vi "Coord Straight Line Move.vi"() -> ()   [LabVIEW 2014]
uses:
  <vilib>/Motion/plugins/PluginFramework/nismSDIFramework.SetFrameworkMode.single.vi
  <vilib>/Motion/PropertyNodes/nimc.createStraightLineMoveInstance.coordinate.vi
  <vilib>/Motion/PropertyNodes/nimc.destroyInterfaceInstance.vi
  <resource>/objmgr/nimotion.rc
  SDI Plug-in - Delta ASDA.lvclass
panel:
  in  "Axis 2":refnum<k21>="Axis 2"
  in  "Axis":refnum<k21>="Axis 1"
  in  "Coordinate Space":refnum<k21>="Coordinate Space 1"
  in  "Position":dbl[](array[numeric])=[1000.0, 2000.0]
  in  "Move Mode":i32(ring)=10551344 items=["Absolute"=10551337, "Relative"=10551344, "Relative To Capture"=10551345, "Velocity"=10551346]
  in  "Acceleration":dbl=10000.0
  in  "Velocity":dbl=1000.0
  out "error out":errorcluster
  out "?":T1(graph)
  in  "Stop Move":bool
  in  "Start Move":bool
  in  "stop":bool
  # "Notes: \n1. This example uses preconfigured settings that may not be appropriate for your motion system. Review and update the axis settings using the Axis Configuration dialog box. Right-click each axis and select Properties to open the Axis Configuration dialog box. \n2. Running this example automatically activates all axes. Disable the \"Enable Drive on Transition to Active Mode\" option on the General Settings page of the Axis Configuration dialog box to prevent axes from activating when the VI runs.\n3. This example uses the default smoothing value to automatically calculate deceleration and jerk values. To specify these move constraints, add them to the move property node.\n\nFor information about using this example in an actual motion system, refer to ni.com/info and enter Info Code nismex."
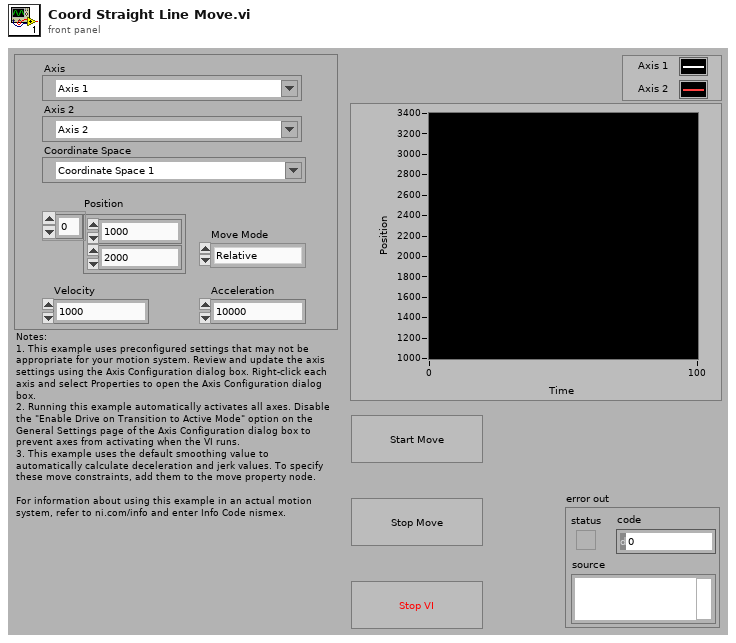
[diagram p1: front panel]
types:
  T1 = cluster{"Commanded Pos.[][0]":dbl, "Commanded Pos.[][1]":dbl}
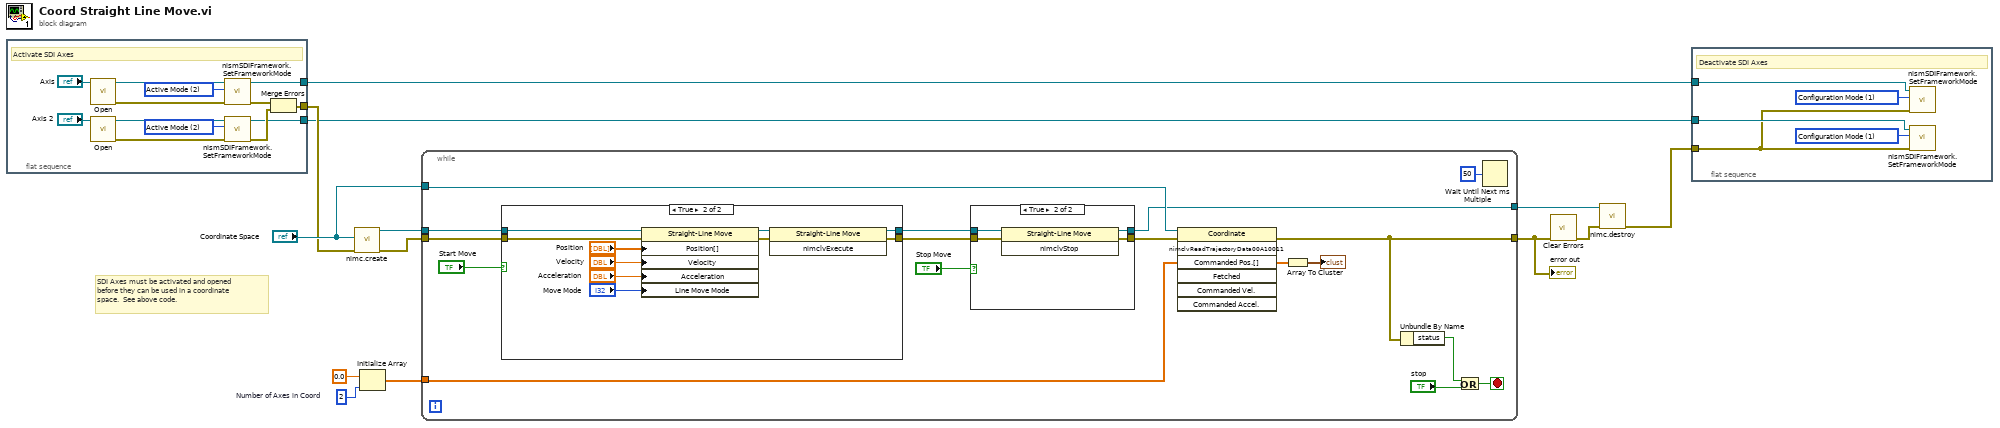
[diagram p0: block diagram]
diagram:
  w6 = 2  # Number of Axes in Coord
  # "SDI Axes must be activated and opened\nbefore they can be used in a coordinate\nspace.  See above code."
  n1 = flat-sequence {
    tunnel: [w16] -> w4
    tunnel: [w15] -> w3
    tunnel: [w14] -> w2
    frame #0 {
      w19 = 2 items=["Configuration Mode"=1, "Active Mode"=2] ("mode (Active Mode)")
      w26 = 2 items=["Configuration Mode"=1, "Active Mode"=2] ("mode (Active Mode)")
      # "Activate SDI Axes"
      n2 = call "Open.vi"("Axis"="Axis") -> ("error out"=w24:errorcluster, "Base Axis Out"=w25:refnum<class "nismPluginAxisBaseClass.lvclass">)  [unwired: 9 in]
      n3 = call "Open.vi"("Axis"="Axis 2") -> ("error out"=w21:errorcluster, "Base Axis Out"=w20:refnum<class "nismPluginAxisBaseClass.lvclass">)  [unwired: 9 in]
      n4 = call-poly <vilib>:"nismSDIFramework.SetFrameworkMode.vi"("error in (no error)"=w24, "mode (Active Mode)"=w26, "Base Axis In"=w25) -> ("error out"=w18:errorcluster, "Base Axis Out"=w15:refnum<class "nismPluginAxisBaseClass.lvclass">)  [unwired: 7 in]
      n5 = call-poly <vilib>:"nismSDIFramework.SetFrameworkMode.vi"("error in (no error)"=w21, "mode (Active Mode)"=w19, "Base Axis In"=w20) -> ("error out"=w17:errorcluster, "Base Axis Out"=w14:refnum<class "nismPluginAxisBaseClass.lvclass">)  [unwired: 7 in]
      n6 = Merge Errors(w18, w17) -> (w16:errorcluster)
    }
  }
  n7 = call-poly <vilib>:"nimc.create.vi"("error in"=w4, "coordinate"="Coordinate Space") -> ("error out"=w12:errorcluster, "line"=w13:refnum<k20>)  [unwired: 7 in, 1 out]
  n8 = Initialize Array(0.0 ("element"), w6) -> (w5:dbl[])
  n9 = while {
    tunnel: w13 -> [w43]
    tunnel: w12 -> [w42]
    tunnel: "Coordinate Space" -> [w34]
    tunnel: [w31] -> w9
    tunnel: [w30] -> w11
    tunnel: w5 -> [w29]
    stop <- w33 stop-if-true
    n10 = case shown="True" "Start Move" {
      tunnel: w43 -> [w51 w61]
      tunnel: w42 -> [w50 w58]
      tunnel: [w50 w57] -> w37
      tunnel: [w51 w56] -> w36
      frame False {
      }
      frame True {
        n11 = property class="Straight-Line Move"(reference=w61, error in=w58, "Position[]"="Position", "Velocity"="Velocity", "Acceleration"="Acceleration", "Line Move Mode"="Move Mode") -> (reference out=w60:refnum<k20>, error out=w59:errorcluster)
        n12 = invoke class="Straight-Line Move" method="nimclvExecute"(reference=w60, error in=w59) -> (reference out=w56:refnum<k20>, error out=w57:errorcluster)  [unwired: 1 in, 1 out]
      }
    }
    n13 = case shown="True" "Stop Move" {
      tunnel: w37 -> [w45 w48]
      tunnel: w36 -> [w44 w49]
      tunnel: [w45 w47] -> w35
      tunnel: [w44 w46] -> w30
      frame False {
      }
      frame True {
        n14 = invoke class="Straight-Line Move" method="nimclvStop"(reference=w49, error in=w48) -> (reference out=w46:refnum<k20>, error out=w47:errorcluster)  [unwired: 1 in, 1 out]
      }
    }
    n15 = invoke class="Coordinate" method="nimclvReadTrajectoryData00A10011"(reference=w34, error in=w35, "Commanded Pos.[]"=w29) -> (error out=w31:errorcluster, "Commanded Pos.[]"=w28:dbl[])  [unwired: 4 in, 5 out]
    n16 = Array To Cluster(array=w28) -> (cluster=→"?":T1)
    n17 = Unbundle By Name(w31) -> ("status"=w32:bool)
    n18 = Or(x=w32, y="stop") -> (x .or. y?=w33:bool)
    n19 = Wait Until Next ms Multiple(millisecond multiple=u32 50 ("milliseconds to wait")) -> ()  [unwired: 1 out]
  }
  "error out" <- w9
  n20 = call <vilib>:"Clear Errors.vi"("error in (no error)"=w9) -> ("error out"=w10:errorcluster)  [unwired: 5 in, 1 out]
  n21 = call-poly <vilib>:"nimc.destroy.vi"("error in"=w10, "motion handle"=w11) -> ("error out"=w1:errorcluster)  [unwired: 9 in]
  n22 = flat-sequence {
    tunnel: w3 -> [w64]
    tunnel: w2 -> [w63]
    tunnel: w1 -> [w62]
    frame #0 {
      w65 = 1 items=["Configuration Mode"=1, "Active Mode"=2] ("mode (Active Mode)")
      w66 = 1 items=["Configuration Mode"=1, "Active Mode"=2] ("mode (Active Mode)")
      # "Deactivate SDI Axes"
      n23 = call-poly <vilib>:"nismSDIFramework.SetFrameworkMode.vi"("error in (no error)"=w62, "mode (Active Mode)"=w66, "Base Axis In"=w64) -> ()  [unwired: 7 in, 2 out]
      n24 = call-poly <vilib>:"nismSDIFramework.SetFrameworkMode.vi"("error in (no error)"=w62, "mode (Active Mode)"=w65, "Base Axis In"=w63) -> ()  [unwired: 7 in, 2 out]
    }
  }
